vi "ObtainVisQueue.vi"(11 "VisualizeBase_class in":refnum<class "VisualizeBase_class.lvclass">) -> (3 "VisualizeBase_class out":refnum<class "VisualizeBase_class.lvclass">)   [LabVIEW 2014, in "Visualization.lvlib" / "VisualizeBase_class.lvclass"]
uses:
  VisializeBase_class/VisualizeBase_class.lvclass
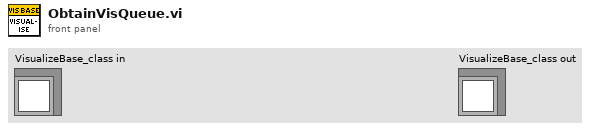
[diagram p1: front panel]
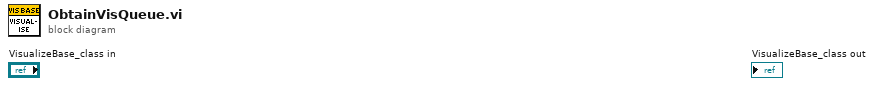
[diagram p0: block diagram]
diagram:
